vi "find mapping by GUID.vi"(10 "owner ID":string, 11 "module Mappings":T1[](array[typedef])) -> (2 "index":i32, 3 "module Mappings out":T1[](array[typedef]))   [LabVIEW 2013, in "engine configuration.lvclass"]
uses:
  engine configuration.lvclass
  Module Mappings.ctl
  <vilib>/NI/Tag Bus/table/mapping specification.ctl
  <vilib>/NI/Tag Bus/tag/Data Type.ctl
  <vilib>/NI/Tag Bus/table/mapping.ctl
  <vilib>/NI/Tag Bus/tag/tag descriptor.lvclass
  <vilib>/NI/Tag Bus/table/data table.lvlib
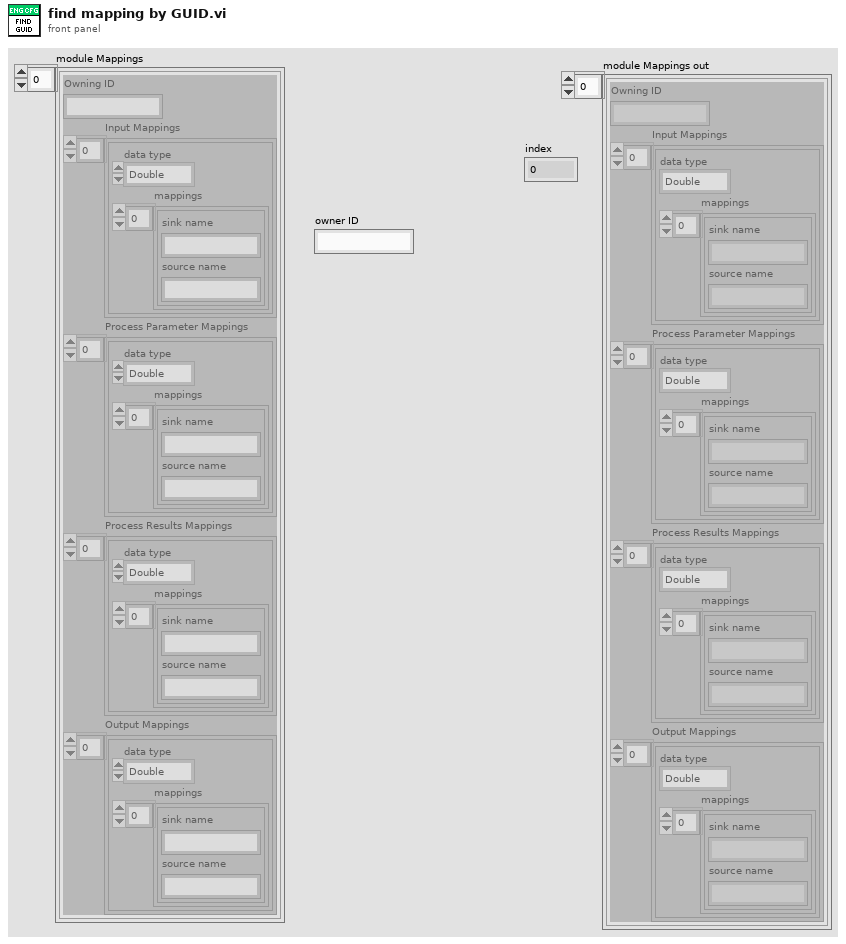
[diagram p1: front panel]
types:
  T1 = typedef "engine configuration.lvclass/Module Mappings.ctl" = cluster{"Owning ID":string, "Input Mappings":T2[], "Process Parameter Mappings":T2[], "Process Results Mappings":T2[], "Output Mappings":T2[]}
  T2 = typedef "tag bus.lvlib/data table.lvlib/mapping specification.ctl" = cluster{"data type":T3, "mappings":T4[]}
  T3 = typedef "tag bus.lvlib/tag descriptor.lvclass/Data Type.ctl" = enum16{"Double", "Single", "I64", "I32", "I16", "I8", "U64", "U32", "U16", "U8", "Boolean", "String", "Array of Double", "Array of Single", "Array of I64", "Array of I32", "Array of I16", "Array of I8", "Array of U64", "Array of U32", "Array of U16", "Array of U8", "Array of Boolean", "Array of String"}
  T4 = typedef "tag bus.lvlib/data table.lvlib/mapping.ctl" = cluster{"sink name":string, "source name":string}
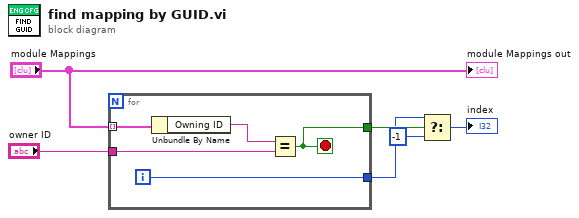
[diagram p0: block diagram]
diagram:
  n1 = for {
    tunnel: "module Mappings" -> [w11] mode=indexing
    tunnel: "owner ID" -> [w10]
    tunnel: [w9] -> w4
    tunnel: [w8] -> w5
    i -> [w9]
    stop <- w8 stop-if-true
    n2 = Unbundle By Name(w11) -> ("Owning ID"=w7:string)
    n3 = Equal?(x=w7, y=w10) -> (x = y?=w8:bool)
  }
  n4 = Select(t=w4, s=w5, f=-1) -> (s? t:f=→"index":i32)
  "module Mappings out" <- "module Mappings"
